vi "HRV_EEG_per_icon.vi"(8 "Icon Number":i32=1, 10 "Trial_Number":i32=1, 11 "ERP_Total":path) -> (3 "Icon1":dbl[][](graph))   [LabVIEW 2014]
uses:
  <vilib>/Utility/file.llb/Read From Spreadsheet File (DBL).vi
panel:
  out "size(s)":i32[](array[numeric])
  in  "index (row)":i32
  out "Icon1 2":dbl[](graph)
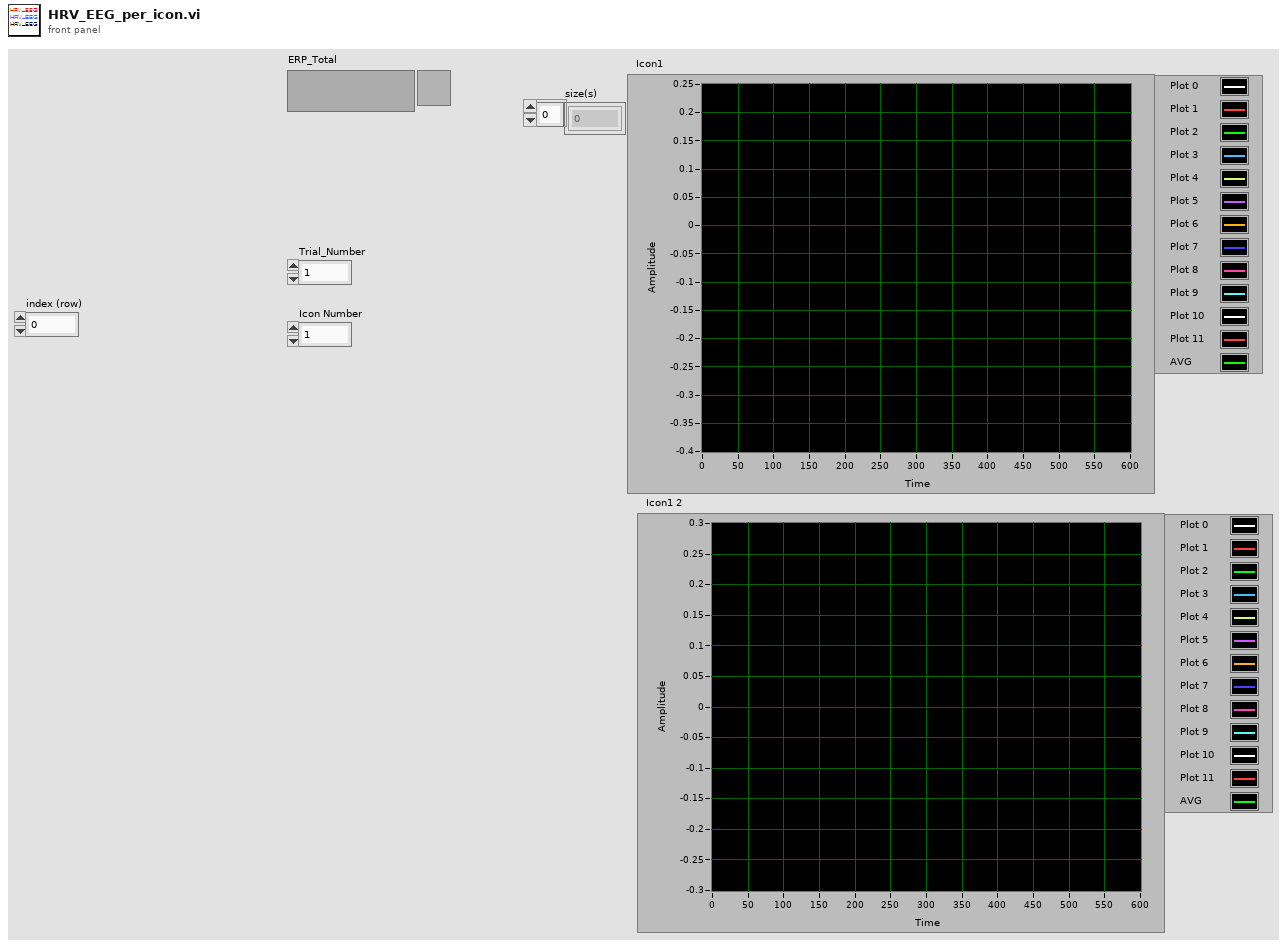
[diagram p1: front panel]
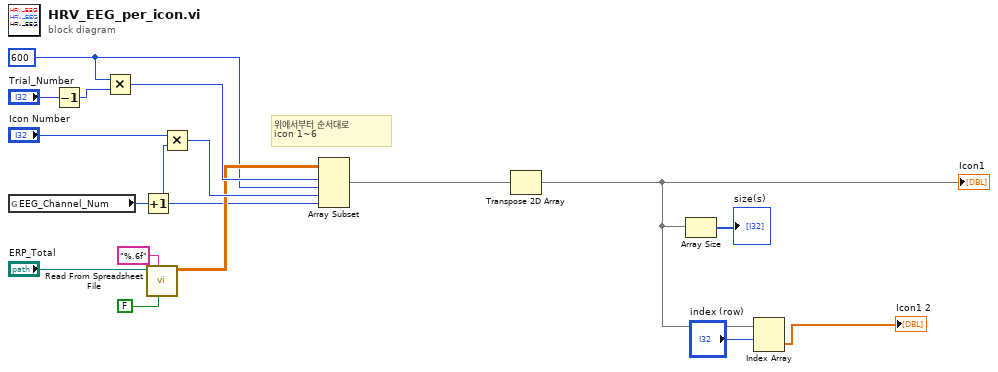
[diagram p0: block diagram]
diagram:
  w8 = 600
  # "위에서부터 순서대로 \nicon 1~6"
  n1 = global read "Control_Panel.vi" "EEG_Channel_Num"() -> (w7:i32)
  n2 = Decrement(x="Trial_Number") -> (x-1=w13:i32)
  n3 = Multiply(x=w8, y=w13) -> (x*y=w15:i32)
  n4 = Increment(x=w7) -> (x+1=w5:i32)
  n5 = call-poly <vilib>:"Read From Spreadsheet File.vi"("transpose (no:F)"=FALSE, "format (%.3f)"="%.6f", "file path (dialog if empty)"="ERP_Total") -> ("all rows"=w9:dbl[][])  [unwired: 4 in, 4 out]
  n6 = Multiply(x="Icon Number", y=w5) -> (x*y=w12:i32)
  n7 = Array Subset(array=w9, index (row)=w15, length (row)=w8, index (col)=w12, length (col)=w5) -> (w6:dbl[][])
  n8 = Transpose 2D Array(2D array=w6) -> (transposed array=w2:dbl[][])
  "Icon1" <- w2
  n9 = Array Size(array=w2) -> (size(s)=→"size(s)":i32[])
  n10 = Index Array(array=w2, index (row)="index (row)") -> (element=→"Icon1 2":dbl[])  [unwired: 1 in]
